vi "TrafficLight_Init.vi"(0 "object in":refnum<class "TrafficLight.lvclass">, 5 "Error In":errorcluster) -> (14 "object out":refnum<class "TrafficLight.lvclass">, 19 "Error Out":errorcluster)   [LabVIEW 2024, in "TrafficLight.lvclass"]
uses:
  TrafficLight.lvclass
  RedState_class/RedState.lvclass
panel:
  # "Connector Pane"
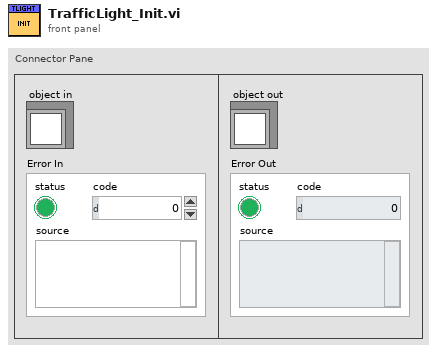
[diagram p1: front panel]
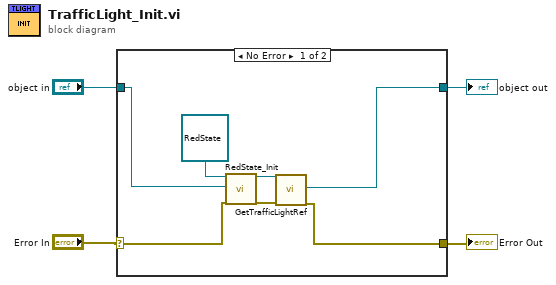
[diagram p0: block diagram]
diagram:
  n1 = case shown="No Error" "Error In" {
    selector: "Error In" -> [w11 w12]
    tunnel: "object in" -> [w9 w13]
    tunnel: [w5 w13] -> w3
    tunnel: [w6 w12] -> w1
    frame No Error {
      n2 = call "RedState_Init.vi"("object in"=refnum<class "RedState.lvclass"> refnum ("RedState"), "TrafficLight"=w9, "Error In"=w11) -> ("object out"=w7:refnum<class "RedState.lvclass">, "Error Out"=w8:errorcluster)  [unwired: 15 in]
      n3 = call-dynamic "GetTrafficLightRef.vi"("object in"=w7, "Error In"=w8) -> ("TrafficLightRef"=w5:refnum<class "TrafficLight.lvclass">, "Error Out"=w6:errorcluster)  [unwired: 15 in, 1 out]
    }
    frame Error {
    }
  }
  "object out" <- w3
  "Error Out" <- w1
